vi "Shooter Control Logic.vi"(9 "Bump Down Flywheel Speed":bool, 10 "Bump Up Flywheel Speed":bool, 11 "Toggle Shooter In":bool) -> (2 "Shooter Speed Calibration":dbl, 3 "Commanded Shooter Speed":dbl, 5 "Toggle Shooter Out":bool)   [LabVIEW 2016]
uses:
  <vilib>/Rock Robotics/WPI/DriverStation/WPI_DriverStationRobotMode2.ctl
  Robot Global Data.vi
  Global Variables/Robot Status.vi
  Global Variables/Shooter Calibrations.vi
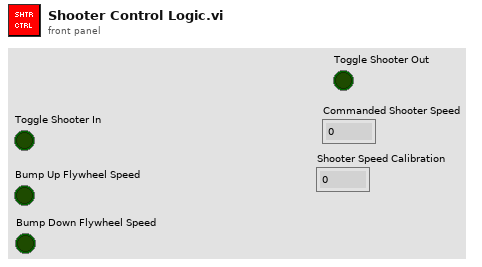
[diagram p1: front panel]
types:
  T1 = typedef "WPI_DriverStationRobotMode2.ctl" = enum16{"Autonomous Disabled", "Autonomous Enabled", "Teleop Disabled", "Teleop Enabled", "Disconnected", "Finish", "Test Disabled", "Test Enabled", "Emergency Stopped"}
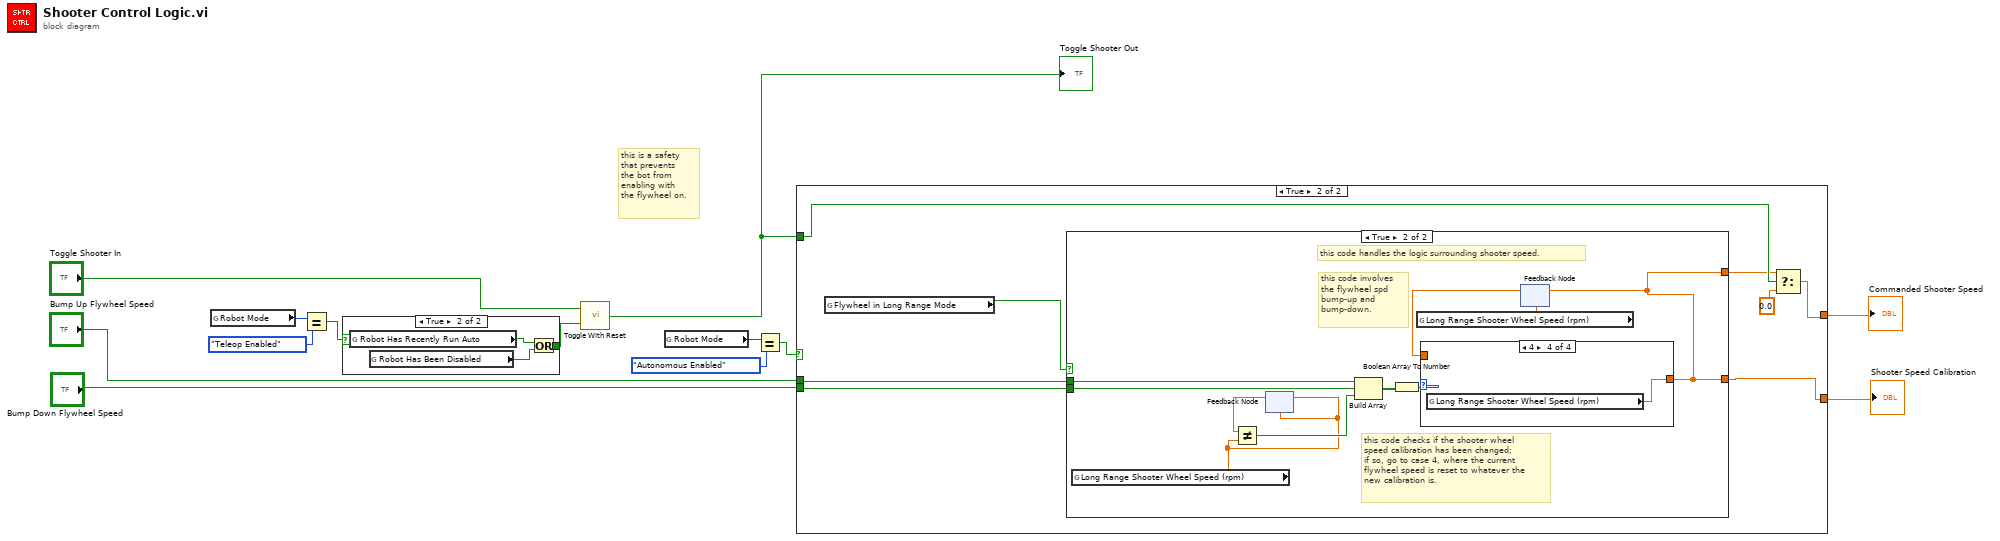
[diagram p0: block diagram]
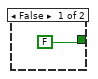
[diagram p2: hidden frame]
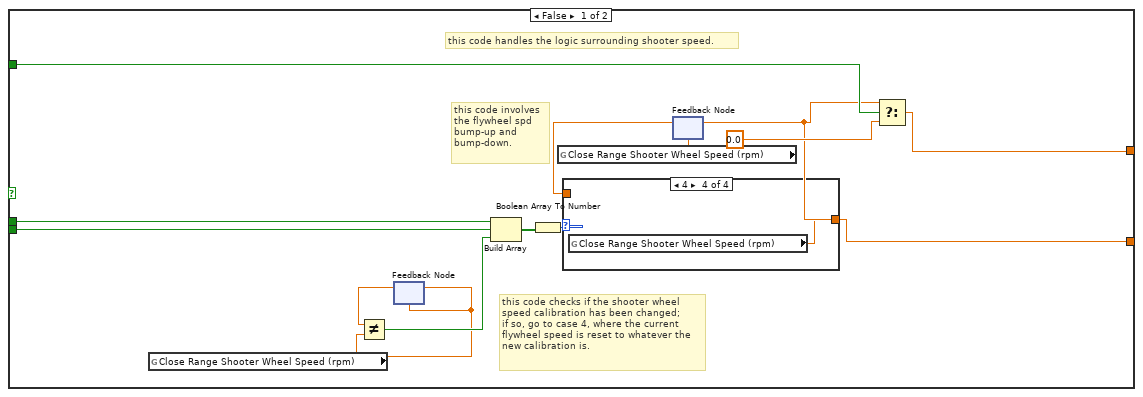
[diagram p3: hidden frame]
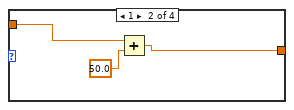
[diagram p5: hidden frame]
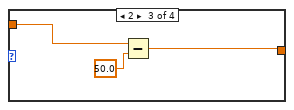
[diagram p6: hidden frame]
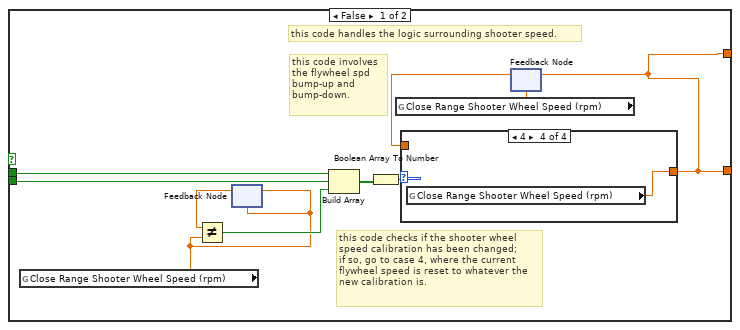
[diagram p7: hidden frame]
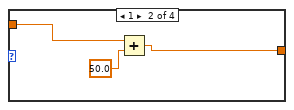
[diagram p9: hidden frame]
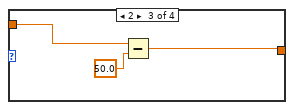
[diagram p10: hidden frame]
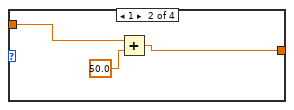
[diagram p12: hidden frame]
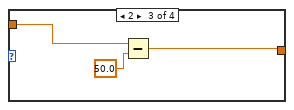
[diagram p13: hidden frame]
diagram:
  # "this is a safety\nthat prevents\nthe bot from\nenabling with\nthe flywheel on."
  n1 = global read "Robot Global Data.vi" "Robot Mode"() -> (w3:T1)
  n2 = Equal?(x=w3, y=WPI_DriverStationRobotMode2."Teleop Enabled" ("Robot Mode")) -> (x = y?=w2:bool)
  n3 = case shown="True" w2 {
    tunnel: [FALSE w15] -> w4
    frame False {
    }
    frame True {
      n4 = global read "Robot Status.vi" "Robot Has Recently Run Auto"() -> (w17:bool)
      n5 = global read "Robot Status.vi" "Robot Has Been Disabled"() -> (w16:bool)
      n6 = Or(x=w17, y=w16) -> (x .or. y?=w15:bool)
    }
  }
  n7 = call "Toggle With Reset.vi"("Reset"=w4, "Boolean"="Toggle Shooter In") -> ("Driver Switch 2"=w10:bool)
  "Toggle Shooter Out" <- w10
  n8 = global read "Robot Global Data.vi" "Robot Mode"() -> (w8:T1)
  n9 = Equal?(x=w8, y=WPI_DriverStationRobotMode2."Autonomous Enabled" ("Robot Mode")) -> (x = y?=w7:bool)
  n10 = case shown="True" w7 {
    tunnel: "Bump Up Flywheel Speed" -> [w29 w44]
    tunnel: "Bump Down Flywheel Speed" -> [w28 w43]
    tunnel: w10 -> [w27 w45]
    tunnel: [w19 w42] -> w6
    tunnel: [w18 w40] -> w5
    frame False {
      # "this code checks if the shooter wheel\nspeed calibration has been changed;\nif so, go to case 4, where the current\nflywheel speed is reset to whatever the\nnew calibration is."
      # "this code involves\nthe flywheel spd\nbump-up and\nbump-down."
      # "this code handles the logic surrounding shooter speed."
      n11 = global read "Shooter Calibrations.vi" "Close Range Shooter Wheel Speed (rpm)"() -> (w20:dbl)
      n12 = feedback #1(w20) -> (w21:dbl)
      n13 = Not Equal?(x=w21, y=w20) -> (x != y?=w22:bool)
      n14 = feedback-in #1(w20) -> ()
      n15 = Build Array(w29, w28, w22) -> (w26:bool[])
      n16 = Boolean Array To Number(Boolean array=w26) -> (number=w25:u32)
      n17 = global read "Shooter Calibrations.vi" "Close Range Shooter Wheel Speed (rpm)"() -> (w23:dbl)
      n18 = feedback #2(w23) -> (w24:dbl)
      n19 = case shown="4" w25 {
        tunnel: w24 -> [w31 w33 w37 _]
        tunnel: [w31 w32 w35 w38] -> w18
        frame 0, Default {
        }
        frame 1 {
          n20 = Add(x=w33, y=50.0) -> (x+y=w32:dbl)
        }
        frame 2 {
          n21 = Subtract(x=w37, y=50.0) -> (x-y=w35:dbl)
        }
        frame 4 {
          n22 = global read "Shooter Calibrations.vi" "Close Range Shooter Wheel Speed (rpm)"() -> (w38:dbl)
        }
      }
      n23 = feedback-in #2(w18) -> ()
      n24 = Select(t=w18, s=w27, f=0.0) -> (s? t:f=w19:dbl)
    }
    frame True {
      n25 = global read "Robot Status.vi" "Flywheel in Long Range Mode"() -> (w39:bool)
      n26 = case shown="True" w39 {
        tunnel: w44 -> [w49 w67]
        tunnel: w43 -> [w48 w66]
        tunnel: [w47 w65] -> w41
        tunnel: [w47 w65] -> w40
        frame False {
          # "this code checks if the shooter wheel\nspeed calibration has been changed;\nif so, go to case 4, where the current\nflywheel speed is reset to whatever the\nnew calibration is."
          # "this code involves\nthe flywheel spd\nbump-up and\nbump-down."
          # "this code handles the logic surrounding shooter speed."
          n27 = global read "Shooter Calibrations.vi" "Close Range Shooter Wheel Speed (rpm)"() -> (w50:dbl)
          n28 = feedback #3(w50) -> (w51:dbl)
          n29 = Not Equal?(x=w51, y=w50) -> (x != y?=w52:bool)
          n30 = feedback-in #3(w50) -> ()
          n31 = Build Array(w49, w48, w52) -> (w56:bool[])
          n32 = Boolean Array To Number(Boolean array=w56) -> (number=w55:u32)
          n33 = global read "Shooter Calibrations.vi" "Close Range Shooter Wheel Speed (rpm)"() -> (w53:dbl)
          n34 = feedback #4(w53) -> (w54:dbl)
          n35 = case shown="4" w55 {
            tunnel: w54 -> [w57 w59 w63 _]
            tunnel: [w57 w58 w61 w64] -> w47
            frame 0, Default {
            }
            frame 1 {
              n36 = Add(x=w59, y=50.0) -> (x+y=w58:dbl)
            }
            frame 2 {
              n37 = Subtract(x=w63, y=50.0) -> (x-y=w61:dbl)
            }
            frame 4 {
              n38 = global read "Shooter Calibrations.vi" "Close Range Shooter Wheel Speed (rpm)"() -> (w64:dbl)
            }
          }
          n39 = feedback-in #4(w47) -> ()
        }
        frame True {
          # "this code checks if the shooter wheel\nspeed calibration has been changed;\nif so, go to case 4, where the current\nflywheel speed is reset to whatever the\nnew calibration is."
          # "this code involves\nthe flywheel spd\nbump-up and\nbump-down."
          # "this code handles the logic surrounding shooter speed."
          n40 = global read "Shooter Calibrations.vi" "Long Range Shooter Wheel Speed (rpm)"() -> (w68:dbl)
          n41 = feedback #5(w68) -> (w69:dbl)
          n42 = Not Equal?(x=w69, y=w68) -> (x != y?=w70:bool)
          n43 = feedback-in #5(w68) -> ()
          n44 = Build Array(w67, w66, w70) -> (w74:bool[])
          n45 = Boolean Array To Number(Boolean array=w74) -> (number=w73:u32)
          n46 = global read "Shooter Calibrations.vi" "Long Range Shooter Wheel Speed (rpm)"() -> (w71:dbl)
          n47 = feedback #6(w71) -> (w72:dbl)
          n48 = case shown="4" w73 {
            tunnel: w72 -> [w75 w77 w81 _]
            tunnel: [w75 w76 w79 w82] -> w65
            frame 0, Default {
            }
            frame 1 {
              n49 = Add(x=w77, y=50.0) -> (x+y=w76:dbl)
            }
            frame 2 {
              n50 = Subtract(x=w81, y=50.0) -> (x-y=w79:dbl)
            }
            frame 4 {
              n51 = global read "Shooter Calibrations.vi" "Long Range Shooter Wheel Speed (rpm)"() -> (w82:dbl)
            }
          }
          n52 = feedback-in #6(w65) -> ()
        }
      }
      n53 = Select(t=w41, s=w45, f=0.0) -> (s? t:f=w42:dbl)
    }
  }
  "Commanded Shooter Speed" <- w6
  "Shooter Speed Calibration" <- w5
